vi "Forloop RNGArray Graph Display.vi"() -> ()   [LabVIEW 2017]
uses:
  <vilib>/Utility/file.llb/Write Delimited Spreadsheet (string).vi
panel:
  out "Time Stamp":timestamp format="%<%.3X>T"
  out "output array":string[][](array[string])
  out "Seconds":i32
  out "Minutes":i32
  out "Hours":i32
  in  "No":bool
  out "Sweep Number":i32
  in  "Yes":bool
  out "First Sweep 2":bool
  in  "?":bool
  in  "Number of Sweeps":i32=1 min=1 max=1000 step=1
  in  "Folder Name":string="Raw Measurement"
  out "Working Folder":path
  in  "Number of Points":i32=10 min=10 max=10000 step=1
  out "Graph":cluster{"Y":dbl[], "Y":dbl[]}[](graph)
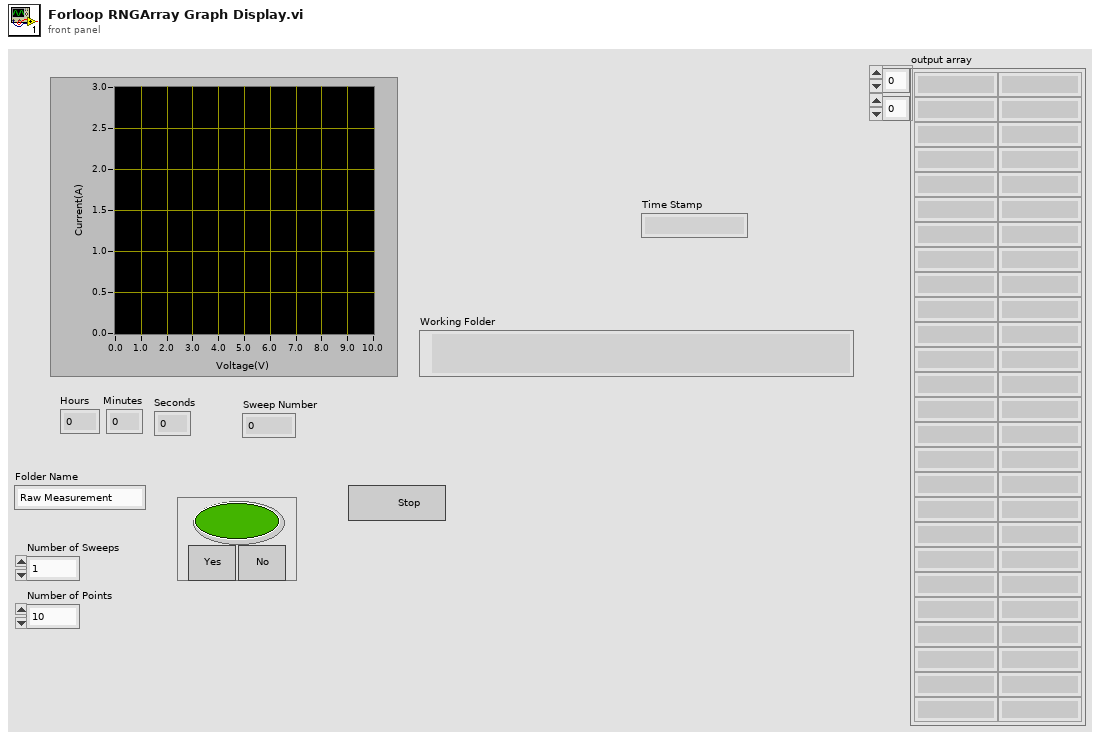
[diagram p1: front panel]
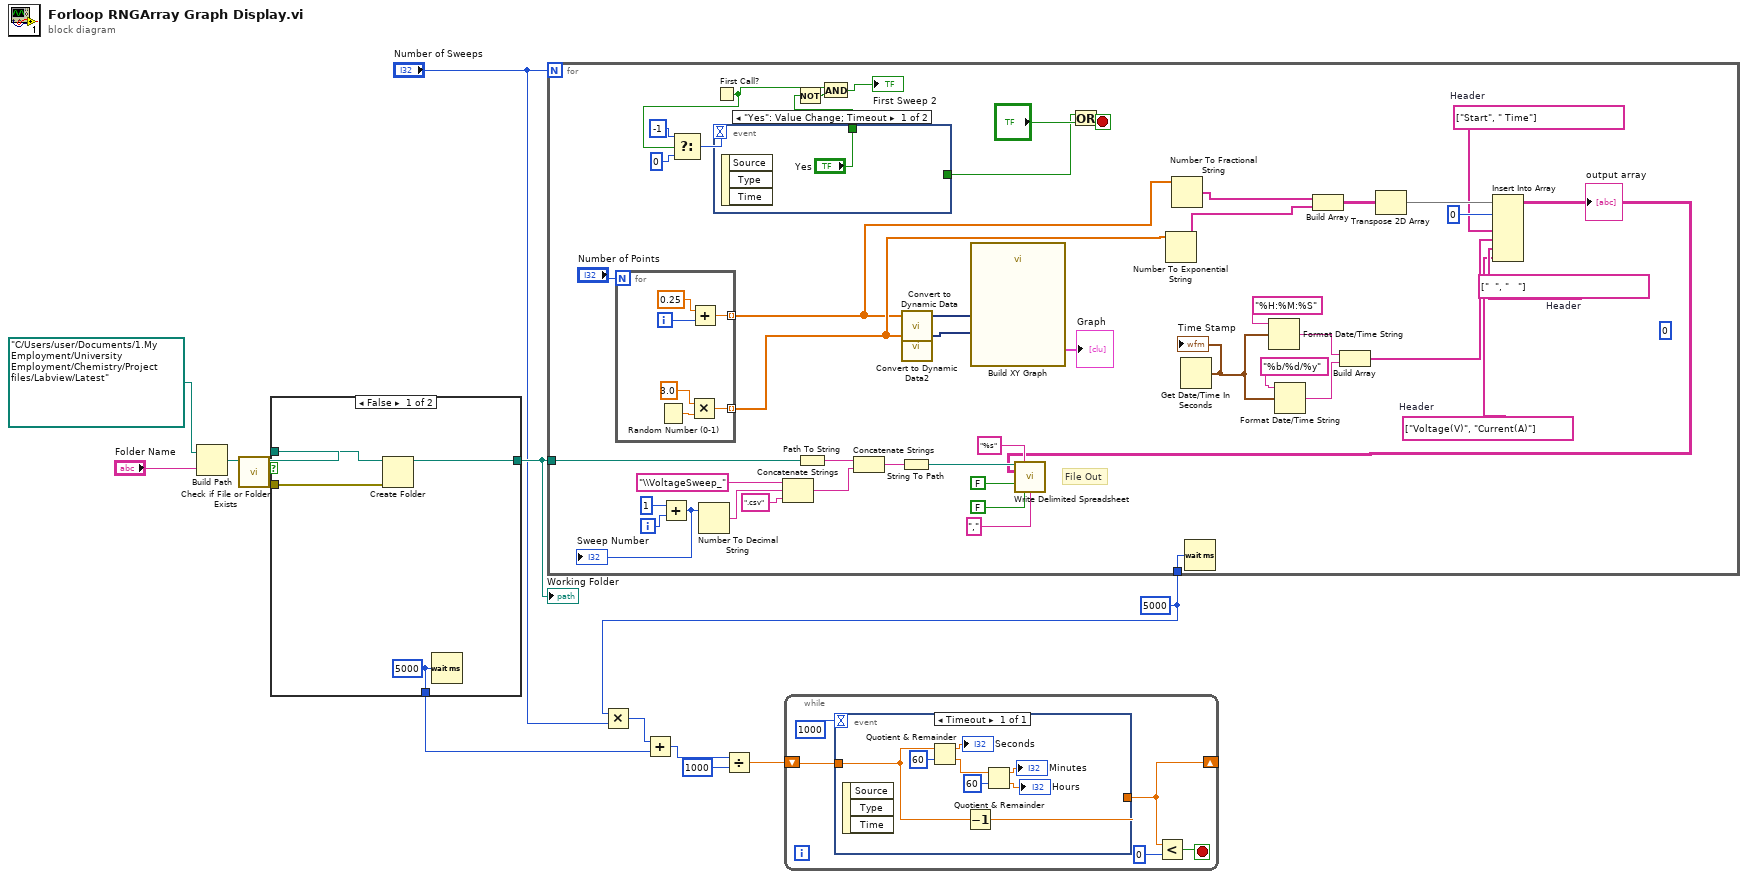
[diagram p0: block diagram]
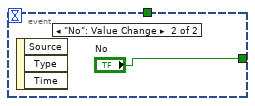
[diagram p2: hidden frame]
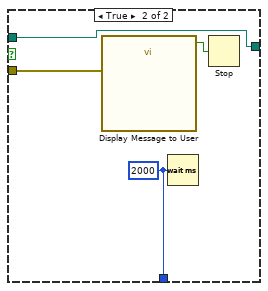
[diagram p3: hidden frame]
diagram:
  w4 = u32 5000 ("milliseconds to wait")
  n1 = Build Path(base path=path "C:/Users/user/Documents/1.My Employment/University Employment/Chemistry/Project files/Labview/Latest" ("Working Directory"), name or relative path="Folder Name") -> (appended path=w12:path)
  n2 = call <vilib>:"Check if File or Folder Exists.vi"("path"=w12) -> ("error out"=w9:errorcluster, "file or folder exists?"=w11:bool, "dup path"=w10:path)  [unwired: 8 in]
  n3 = case shown="False" w11 {
    tunnel: [w17 w20] -> w8
    tunnel: w10 -> [w18 w20]
    tunnel: w9 -> [w16 w22]
    tunnel: [w15 w19] -> w7
    frame False {
      w15 = u32 5000 ("milliseconds to wait")
      n4 = Create Folder(path (use dialog)=w18, error in=w16) -> (created path=w17:path)  [unwired: 1 in, 2 out]
      n5 = Wait (ms)(milliseconds to wait=w15) -> ()  [unwired: 1 out]
    }
    frame True {
      w19 = u32 2000 ("milliseconds to wait")
      n6 = call "Display Message to User"("error in (no error)"=w22) -> ("OK"=w21:bool)  [unwired: 9 in, 1 out]
      n7 = Wait (ms)(milliseconds to wait=w19) -> ()  [unwired: 1 out]
      n8 = Stop(stop? (T)=w21) -> ()
    }
  }
  "Working Folder" <- w8
  n9 = for {
    N: "Number of Sweeps" -> [_]
    tunnel: w8 -> [w62]
    tunnel: w4 -> [w49]
    i -> [w55]
    stop <- w25 stop-if-true
    w34 = string[] ["  ", "   "]  # Header
    (unwired) 0 ("index (row)")
    w36 = string[] ["Start", " Time"]  # Header
    w33 = string[] ["Voltage(V)", "Current(A)"]  # Header
    # "File Out"
    n10 = for {
      N: "Number of Points" -> [_]
      tunnel: [w73] -> w31 mode=indexing
      tunnel: [w72] -> w44 mode=indexing
      i -> [w74]
      n11 = Random Number (0-1)() -> (number: 0 to 1=w75:dbl)
      n12 = Multiply(x=3.0, y=w75) -> (x*y=w72:dbl)
      n13 = Add(x=0.25 ("y"), y=w74) -> (x+y=w73:dbl)
    }
    n14 = Add(x=1, y=w55) -> (x+y=w50:i32)
    "Sweep Number" <- w50
    n15 = Number To Decimal String(number=w50) -> (decimal integer string=w53:string)  [unwired: 1 in]
    n16 = First Call?() -> (First Call?: T/F=w29:bool)
    n17 = Select(t=-1, s=w29, f=0) -> (s? t:f=w51:i32)
    n18 = event shown="[0] \"Yes\": Value Change;  Timeout" {
      selector: _ -> [_ _]
      dyn-events: _ -> [_ _]
      timeout: w51 -> [_ _]
      tunnel: [_ "No"] -> w24
      tunnel: ["Yes" _] -> w23
      event "Yes": Value Change; Timeout {
        n19 = event-data() -> ()  [unwired: 1 in, 3 out]
      }
      event "No": Value Change {
        n20 = event-data() -> ()  [unwired: 1 in, 3 out]
      }
    }
    n21 = Concatenate Strings("\\VoltageSweep_" ("string"), w53, ".csv" ("string")) -> (w58:string)
    n22 = Not(x=w23) -> (.not. x?=w27:bool)
    n23 = Path To String(path=w62) -> (string=w64:string)
    n24 = And(x=w29, y=w27) -> (x .and. y?=→"First Sweep 2":bool)
    n25 = Concatenate Strings(w64, w58) -> (w63:string)
    n26 = String To Path(string=w63) -> (path=w48:path)
    n27 = call "Convert to Dynamic Data"("Array"=w31) -> ("Dynamic Data Type"=w69:dynamicdata)  [unwired: 3 in]
    n28 = call "Convert to Dynamic Data2"("Array"=w44) -> ("Dynamic Data Type"=w68:dynamicdata)  [unwired: 3 in]
    n29 = call "Build XY Graph"("Y Input"=w68, "X Input"=w69) -> ("XY Graph"=→"Graph":cluster{"X":dbl[], "Y":dbl[]}[])  [unwired: 8 in, 1 out]
    n30 = Or(x=w24, y="?") -> (x .or. y?=w25:bool)
    n31 = Number To Exponential String(number=w44) -> (E-format string=w42:string[])  [unwired: 3 in]
    n32 = Number To Fractional String(number=w31) -> (F-format string=w43:string[])  [unwired: 3 in]
    n33 = Get Date/Time In Seconds() -> (seconds since 1Jan1904=w37:timestamp)
    "Time Stamp" <- w37
    n34 = Wait (ms)(milliseconds to wait=w49) -> ()  [unwired: 1 out]
    n35 = Format Date/Time String(time format string (%c)="%H:%M:%S", seconds (now)=w37) -> (date/time string=w40:string)  [unwired: 1 out]
    n36 = Format Date/Time String(time format string (%c)="%b/%d/%y", seconds (now)=w37) -> (date/time string=w39:string)  [unwired: 1 out]
    n37 = Build Array(w43, w42) -> (w46:string[][])
    n38 = Build Array(w40, w39) -> (w35:string[])
    n39 = Transpose 2D Array(2D array=w46) -> (transposed array=w47:string[][])
    n40 = Insert Into Array "Insert Into Array"(array=w47, index (row)=0, new element #1=w36, new element #2=w35, new element #3=w34, new element #4=w33) -> (w32:string[][])  [unwired: 1 in]
    "output array" <- w32
    n41 = call-poly <vilib>:"Write Delimited Spreadsheet.vi"("file path (dialog if empty)"=w48, "format (%s)"="%s" ("format (%.3f)"), "2D data"=w32, "append to file? (new file:F)"=FALSE, "transpose? (no:F)"=FALSE, "delimiter (\\t)"="," ("delimiter (\\t)")) -> ()  [unwired: 8 in, 2 out]
  }
  n42 = Multiply(x=w4, y="Number of Sweeps") -> (x*y=w6:u32)
  n43 = Add(x=w6, y=w7) -> (x+y=w3:u32)
  n44 = Divide(x=w3, y=u32 1000) -> (x/y=w1:dbl)
  n45 = while {
    shift-right: [w79] -> _
    shift-left: w1 -> [w81]
    stop <- w80 stop-if-true
    n46 = event shown="[0] Timeout" {
      selector: _ -> [_]
      dyn-events: _ -> [_]
      timeout: 1000 -> [_]
      tunnel: w81 -> [w88]
      tunnel: [w90] -> w79
      event Timeout {
        n47 = event-data() -> ()  [unwired: 1 in, 3 out]
        n48 = Quotient & Remainder(x=w88, y=60) -> (x-y*floor(x/y)=→"Seconds":dbl, floor(x/y)=w84:dbl)
        n49 = Decrement(x=w88) -> (x-1=w90:dbl)
        n50 = Quotient & Remainder(x=w84, y=60) -> (x-y*floor(x/y)=→"Minutes":dbl, floor(x/y)=→"Hours":dbl)
      }
    }
    n51 = Less?(x=w79, y=0) -> (x < y?=w80:bool)
  }
